vi "Convert to Encoded Error Cluster.vi"(11 "error in":errorcluster) -> (3 "error out":errorcluster)   [LabVIEW 2020, in "Multi Error Cluster.lvlib"]
doc: "Converts an error cluster from legacy format to JSON encoded format."
uses:
  <vilib>/MultiError/TokenizeJSON/Multi Error Cluster.lvlib
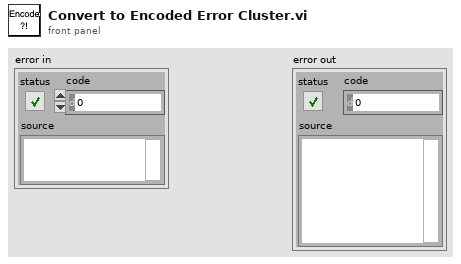
[diagram p1: front panel]
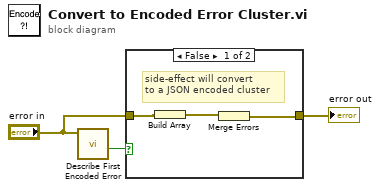
[diagram p0: block diagram]
diagram:
  n1 = call <vilib>:"Describe First Encoded Error.vi"("error in"="error in") -> ("encoded"=w3:bool)  [unwired: 9 in, 1 out]
  n2 = case shown="False" w3 {
    tunnel: "error in" -> [w6 w7]
    tunnel: [w4 w7] -> w1
    frame False {
      # "side-effect will convert\nto a JSON encoded cluster"
      n3 = Build Array(w6) -> (w5:errorcluster[])
      n4 = Merge Errors(w5) -> (w4:errorcluster)
    }
    frame True {
    }
  }
  "error out" <- w1
